vi "ZAlign_MaxPos.vi"(8 "error in (no error)":errorcluster, 10 "Objects":refnum<vi>[](array[refnum]), 11 "Panel":refnum<vi>) -> (0 "error out":errorcluster, 2 "Max right location":u32, 3 "Height":u32)   [LabVIEW 2014, in "ZAlign.lvlib"]
doc: "ZAlign.lvlib:ZAlign_MaxPos.vi\n----------------------------------------------\nGet Max position\n\nInputs:\n---------------------\n- error in (no error) : Cluster; \n- Objects : 1DArrayOfRefnum; \n- Panel : Refnum; \n\nOutputs:\n---------------------\n- error out : Cluster; \n- Max right location : U32; \n- Height : U32; \n\n----------------------------------------------\n16/03/2015\nZühlke Engineering AG\nCH-8952 Schlieren\nwww.zuehlke.com"
uses:
  ZAlign.lvlib
panel:
  out "Width Array":u32[](array[numeric])
  # "Connector Pane"
  # "Locals"
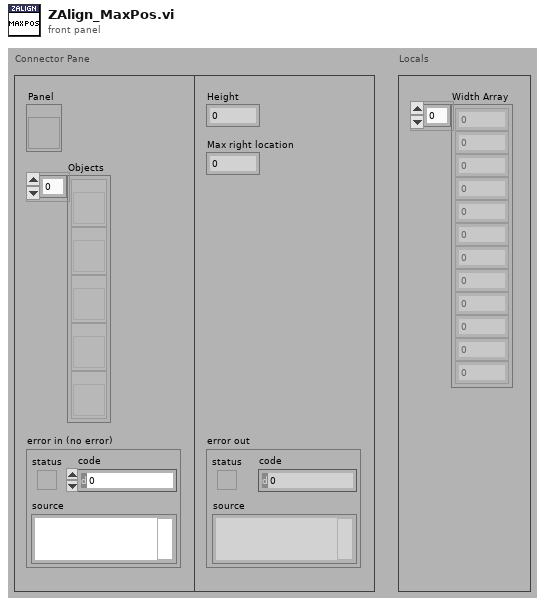
[diagram p1: front panel]
types:
  T1 = typedef "LVPositionTypeDef.ctl" = cluster{"Left":i32, "Top":i32}
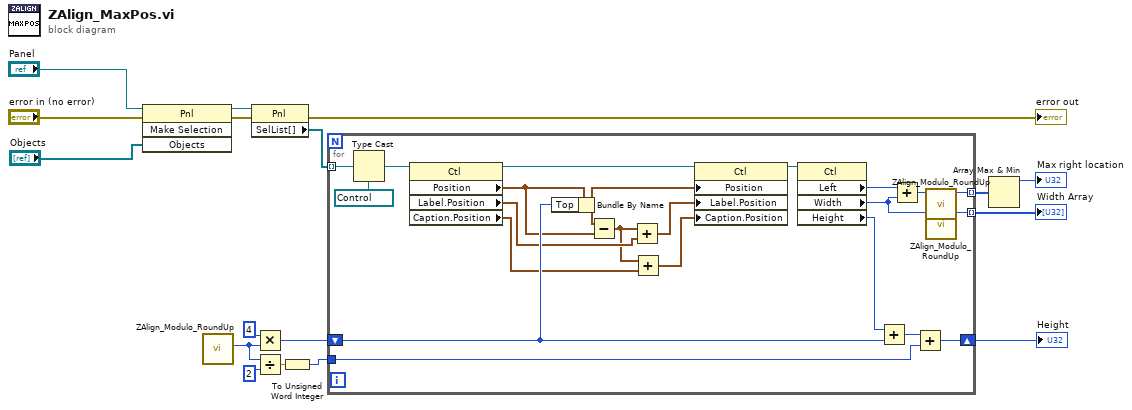
[diagram p0: block diagram]
diagram:
  n1 = invoke class="Pnl" method="Make Selection"(reference="Panel", error in="error in (no error)", "Objects"="Objects") -> (reference out=w8:refnum<vi>, error out=w9:errorcluster)  [unwired: 1 in, 2 out]
  n2 = call "ZAlign_Modulo_RoundUp.vi"() -> ("Grid_Size"=w4:i32)  [unwired: 10 in, 1 out]
  n3 = property class="Pnl"(reference=w8, error in=w9) -> (error out=→"error out":errorcluster, "SelList[]"=w15:refnum<vi>[])  [unwired: 1 out]
  n4 = Multiply(x=i16 4 ("y"), y=w4) -> (x*y=w7:i32)
  n5 = Divide(x=w4, y=i16 2) -> (x/y=w3:dbl)
  n6 = To Unsigned Word Integer(number=w3) -> (unsigned 16bit integer=w2:u16)
  n7 = for {
    tunnel: w15 -> [w30] mode=indexing
    tunnel: [w34] -> w16 mode=indexing
    tunnel: [w32] -> w13 mode=indexing
    shift-right: [w31] -> w1
    shift-left: w7 -> [w25]
    tunnel: w2 -> [w36]
    n8 = Type Cast(type=refnum<vi> refnum ("reference out"), x=w30) -> (*(type *) &x=w28:refnum<vi>)
    n9 = property class="Ctl"(reference=w28) -> (reference out=w27:refnum<vi>, "Position"=w23:T1, "Label.Position"=w21:T1, "Caption.Position"=w19:T1)  [unwired: 1 in, 1 out]
    n10 = Bundle By Name(cluster=w23, "Top"=w25) -> (w24:T1)
    n11 = Subtract(x=w24, y=w23) -> (x-y=w20:T1)
    n12 = Add(x=w20, y=w21) -> (x+y=w22:T1)
    n13 = Add(x=w20, y=w19) -> (x+y=w18:T1)
    n14 = property class="Ctl"(reference=w27, "Position"=w24, "Label.Position"=w22, "Caption.Position"=w18) -> (reference out=w26:refnum<vi>)  [unwired: 1 in, 1 out]
    n15 = property class="Ctl"(reference=w26) -> ("Left"=w39:i32, "Width"=w33:u32, "Height"=w38:u32)  [unwired: 1 in, 2 out]
    n16 = Add(x=w38, y=w25) -> (x+y=w37:u32)
    n17 = Add(x=w39, y=w33) -> (x+y=w35:u32)
    n18 = Add(x=w37, y=w36) -> (x+y=w31:u32)
    n19 = call "ZAlign_Modulo_RoundUp.vi"("Value in"=w35) -> ("Value out"=w34:i32)  [unwired: 9 in, 1 out]
    n20 = call "ZAlign_Modulo_RoundUp.vi"("Value in"=w33) -> ("Value out"=w32:i32)  [unwired: 9 in, 1 out]
  }
  "Width Array" <- w13
  "Height" <- w1
  n21 = Array Max & Min(array=w16) -> (max value=→"Max right location":i32)  [unwired: 3 out]
